vi "Window-Patches acq viewer (experimental).vi"() -> ()   [LabVIEW 2017]
uses:
  User Interface/Visualisation/Timelapse Viewer/Typedefs/Speed Viewer States enum.ctl
  User Interface/Visualisation/Timelapse Viewer/Typedefs/Time series viewer refs.ctl
  User Interface/Visualisation/Timelapse Viewer/Globals/gl_Time series viewer globals.vi
  User Interface/Visualisation/Timelapse Viewer/Typedefs/Select Play-Stop button to show.ctl
  <vilib>/Utility/miscctls.llb/LVPointTypeDef.ctl
  <vilib>/vision/Image Controls.llb/IMAQ Image.ctl
  User Interface/Visualisation/Timelapse Viewer/Cam video sync/Typedefs/Cam videos cluster.ctl
  User Interface/Visualisation/Functional Imaging Viewer/Typedefs/Get-Set-Clear Control.ctl
  <vilib>/Utility/error.llb/DialogType.ctl
  Typedefs/Save-Load enum.ctl
  User Interface/Visualisation/Timelapse Viewer/Typedefs/Custom slider-vertical.ctl
panel:
  in  "Speed chart history (sec)":i32=10
  out "Number of Frames":u32
  in  "Source number of frames":T1(ring)=enum."As many as the number of cycles"
  out "Cams":T3 {"Vid4 Rel time (ms)" format="%.0f ms"; "Vid3 Rel time (ms)" format="%.0f ms"; "Vid2 Rel time (ms)" format="%.0f ms"; "Vid1 Rel time (ms)" format="%.0f ms"}
  out "Original frame rate (fps)":dbl format="Original frame rate: %#.1f (fps)"
  out "Frame rate set (fps)":dbl format="Frame rate set: %#.1f (fps)"
  out "Actual frame rate (fps)":dbl format="Actual frame rate: %#.1f (fps)"
  out "AVI Mode ind":string="AVI mode:"
  out "Video length info":string="Duration: 00h 00m 00s, 0 frames"
  in  "Experiment path":path=path "C:/Users/Teo/Desktop/UCL Datasets/150501_13_00_36 SRINIVAS PATCHES"
  out "Export images":bool
  out "Export snippet":bool
  in  "Extraction Cursors":cluster{i32, i32}(slide)={1, 5594} scale=1.0..1950.0
  out "Export vid":bool
  out "Stop (ind)":bool
  in  "Intensity":T4={0.0, 4095.0} scale=0.0..4095.0
  out "Slider at frame #":i32 format="Slider at time-series frame: %.0f"
  in  "Scrollbar":i32(c297)
  in  "Back":bool
  in  "Play":bool
  in  "Stop":bool
  out "Actual number of speed points":i32 format="Actual of speed points: %.0f"
  out "Speed Data":string[][](array[string])
  out "Expected speed values":dbl format="Expected speed points: %#_g"
  in  "Colour":enum16{"Gray", "Red", "Green"}(ring)
  out "Image":T2(plugin-control)
  out "Speed Graph":dbl[](graph) caption="Speed Chart"
  # "This tool is under development.\nIt currently loads and displays cam videos and speed data acquired during functional acquisition experiments (POI/rectangles/volumes). It may be upgraded to visualise imaging data too."
  # "Timelapse Info"
  # "Date                         Time                  Time stamp           Speed (rpm)          Angle (deg)"
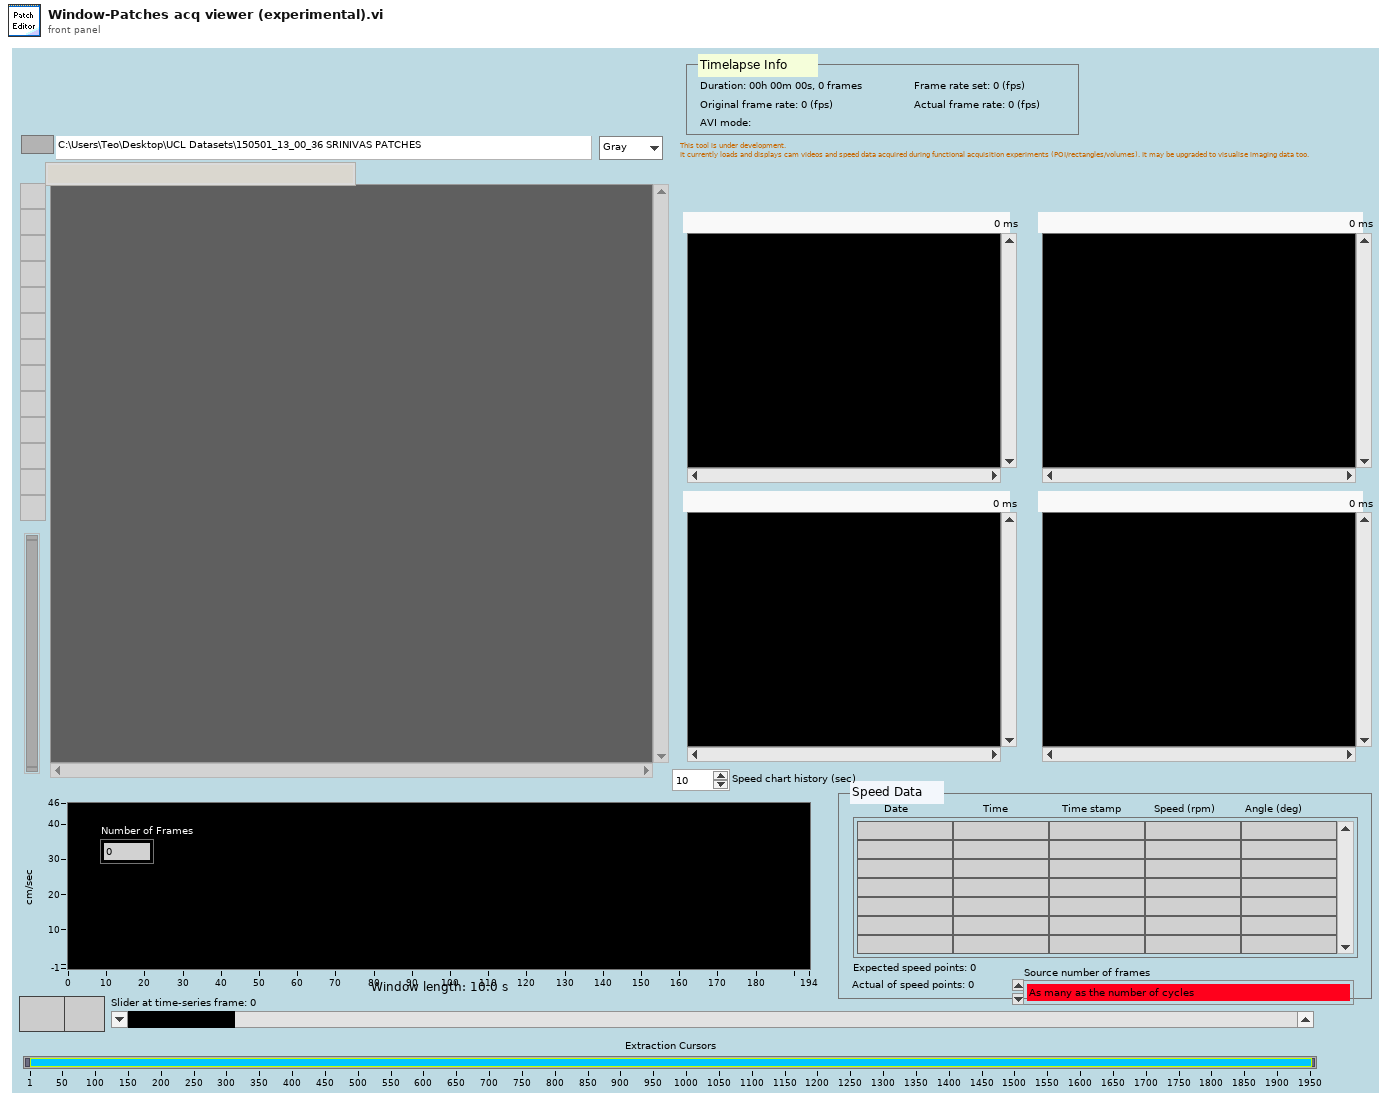
[diagram p1: front panel]
types:
  T1 = enum16{"As many as the frames in the video with the fewest frames", "As many as the number of cycles"}
  T2 = typedef "IMAQ Image.ctl" = refnum<image>
  T3 = cluster{"Vid 1":T2, "Vid 2":T2, "Vid 3":T2, "Vid 4":T2, "Vid1 Rel time (ms)":u32, "Vid2 Rel time (ms)":u32, "Vid3 Rel time (ms)":u32, "Vid4 Rel time (ms)":u32}
  T4 = typedef "Custom slider-vertical.ctl" = cluster{dbl, dbl}
  T5 = typedef "Time series viewer refs.ctl" = cluster{"This VI":refnum<vi>, "Image control":refnum<vi>, "AVI Mode ind":refnum<vi>, "Play":refnum<vi>, "Stop":refnum<vi>, "Back":refnum<vi>, "Scrollbar":refnum<vi>, "Video length info":refnum<vi>, "Expected speed values":refnum<vi>, "Intensity":refnum<vi>, "Path":refnum<vi>, "Selection sliders":refnum<vi>, "Speed Graph ref":refnum<vi>, "Frame rate set (fps)":refnum<vi>, "Channel to load":refnum<vi>, "Number of rows to generate":refnum<vi>, "Colour":refnum<vi>}
  T6 = typedef "Save-Load enum.ctl" = enum16{"Save to file", "Load from file", "Compare from file"}
  T7 = enum16{"None", "Release queue", "Obtain queue", "Enqueue", "Get status", "Set status"}
  T8 = typedef "LVPointTypeDef.ctl" = cluster{"Horizontal":i16, "Vertical":i16}
  T9 = typedef "Speed Viewer States enum.ctl" = enum16{"Idle", "Initialise", "Playback", "Scroll bar event", "Speed cursor event", "Back to start", "Exit"}
  T10 = typedef "Image Type" = u32
  T11 = typedef "IMAQ AVI2 Refnum.ctl" = refnum<k20>
  T12 = cluster{"# of frames to export":i32, "Initial frame's owning file":T11, "8-bit AVI file path":path, "Cursors location":cluster{"Number of first frame":i32, "Number of last frame":i32}}
  T13 = typedef "Get-Set-Clear Control.ctl" = enum16{"Get", "Set", "Clear"}
  T14 = typedef "Select Play-Stop button to show.ctl" = enum16{"Show Play button", "Show Stop button"}
  T15 = typedef "Cam videos cluster.ctl" = cluster{"Vid 1":T2, "Vid 2":T2, "Vid 3":T2, "Vid 4":T2, "Vid1 Rel time (ms)":u32, "Vid2 Rel time (ms)":u32, "Vid3 Rel time (ms)":u32, "Vid4 Rel time (ms)":u32}
  T16 = typedef "DialogType.ctl" = u16
  T17 = typedef "AVI modes refs cluster.ctl" = cluster{"AVI1 ref":T18, "AVI2 refs":T11[], "AVI # frames":u32[]}
  T18 = typedef "AviRefnum.ctl" = refnum<k1>
  T19 = typedef "AVI implementation enum.ctl" = enum16{"AVI1", "AVI2"}
  T20 = enum32{"Invalid", "Standard", "Closed", "Hidden", "Minimized", "Maximized"}
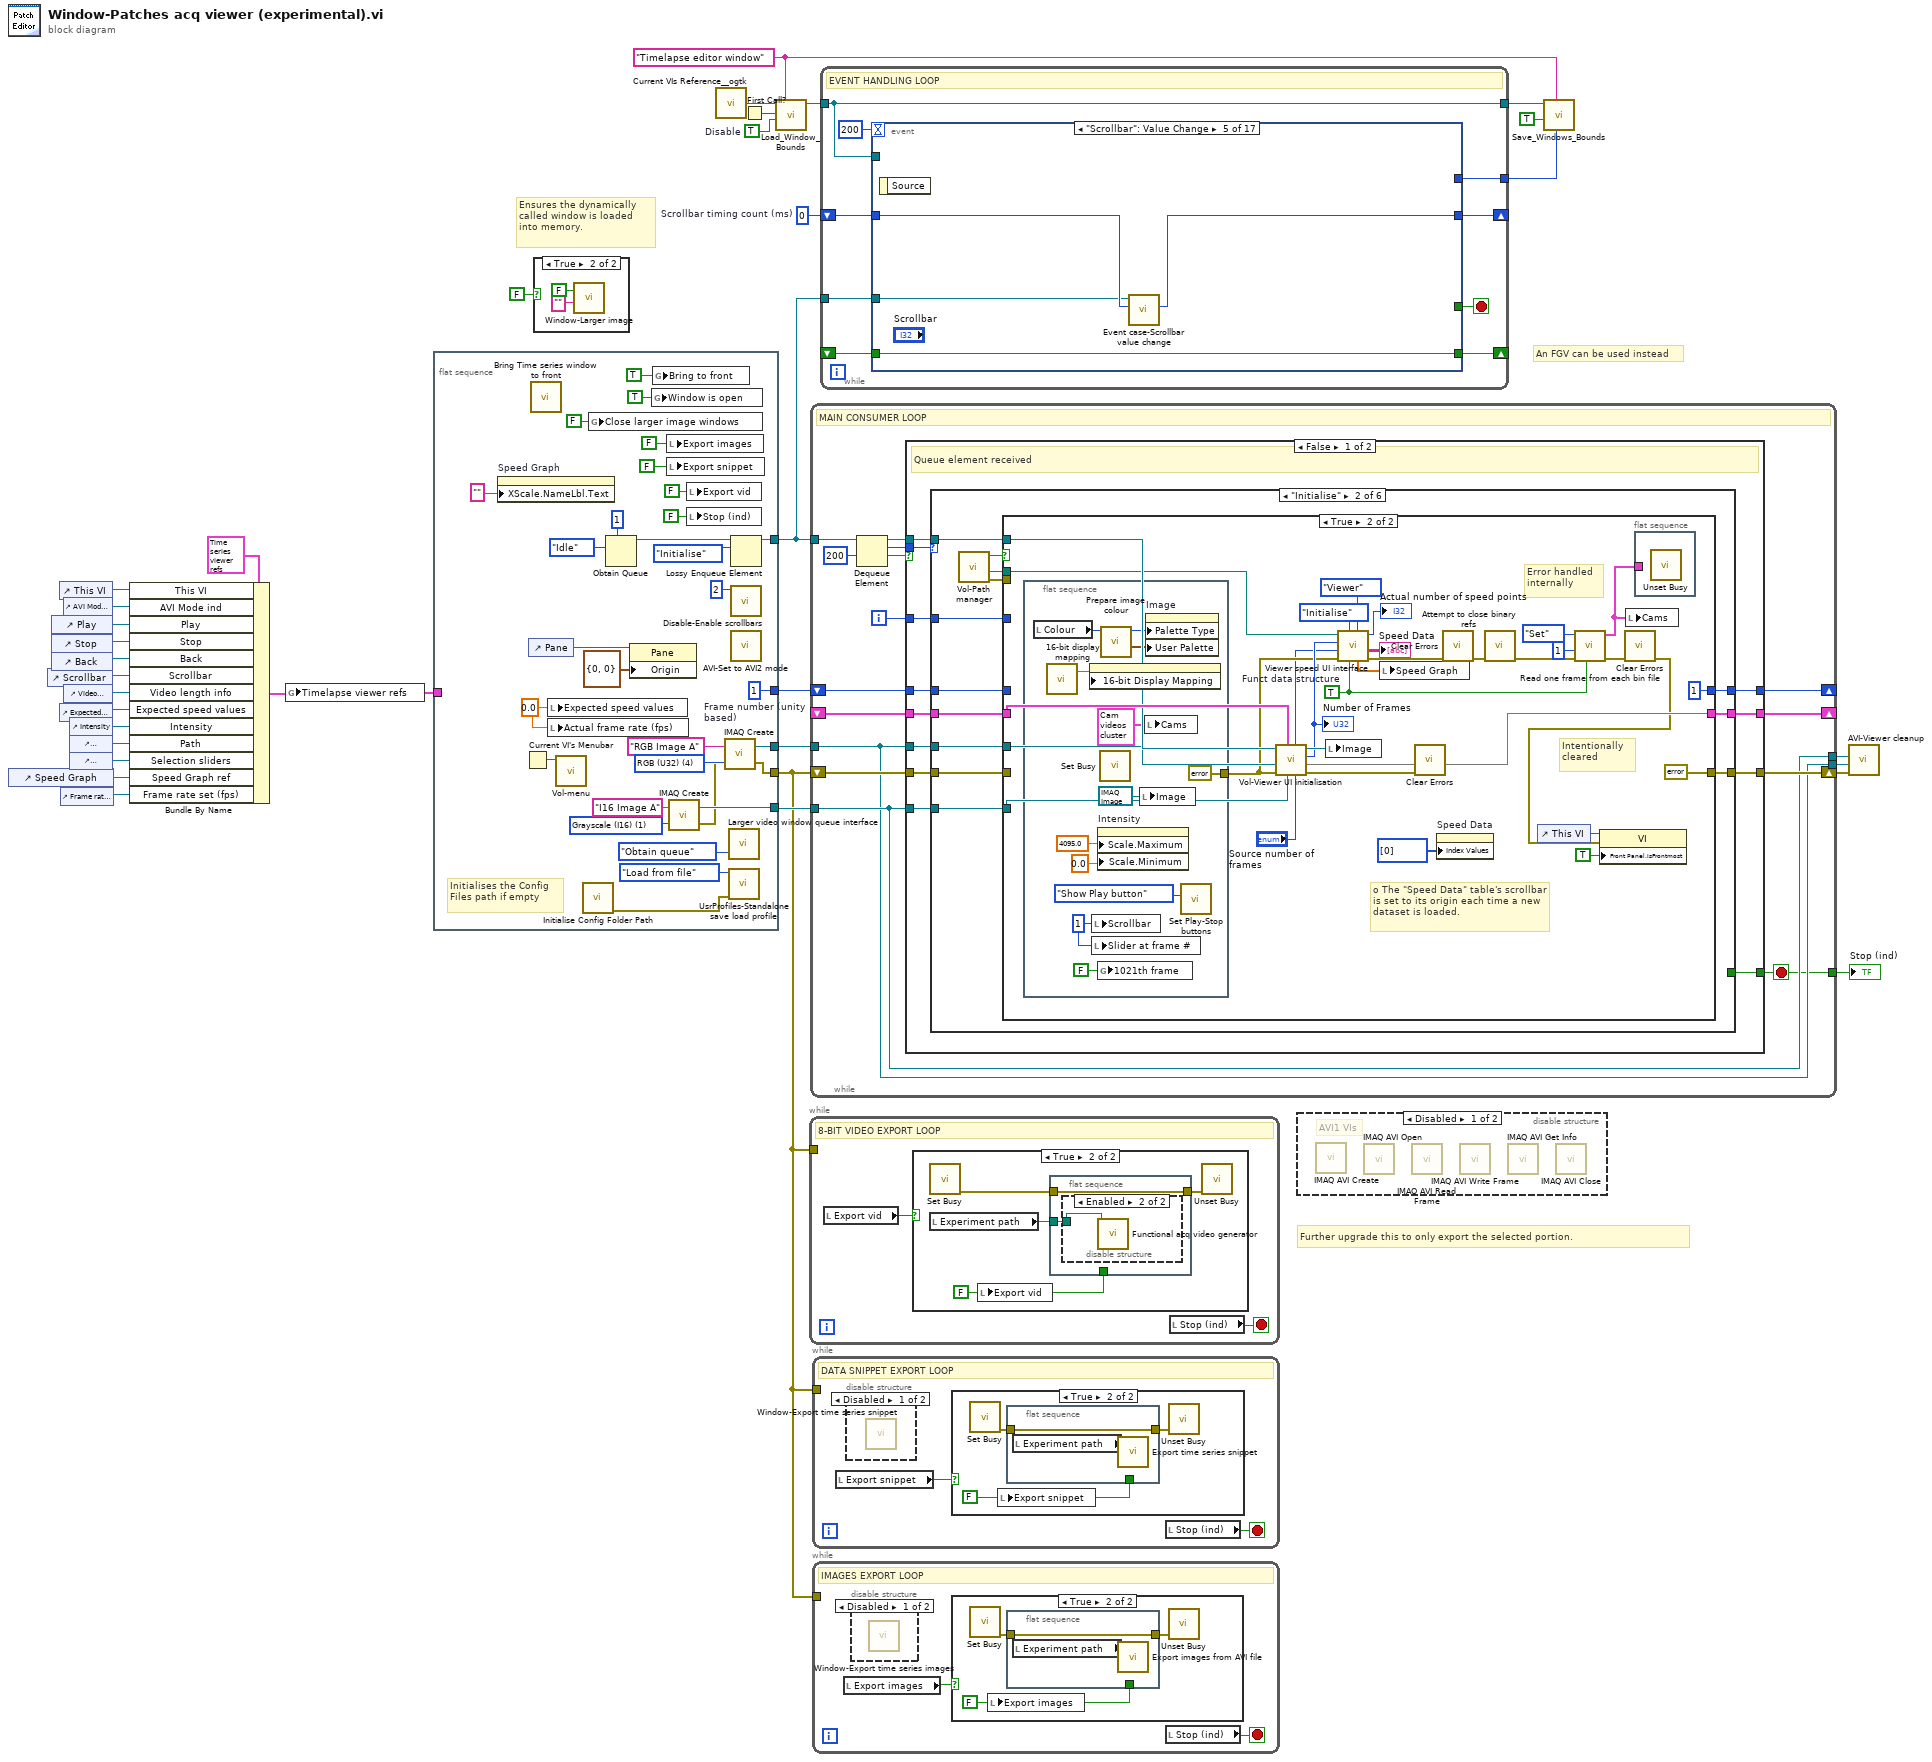
[diagram p0: block diagram]
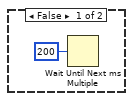
[diagram p4: hidden frame]
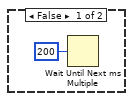
[diagram p6: hidden frame]
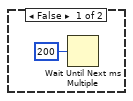
[diagram p8: hidden frame]
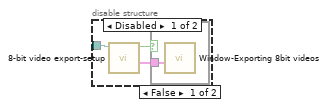
[diagram p9: hidden frame]
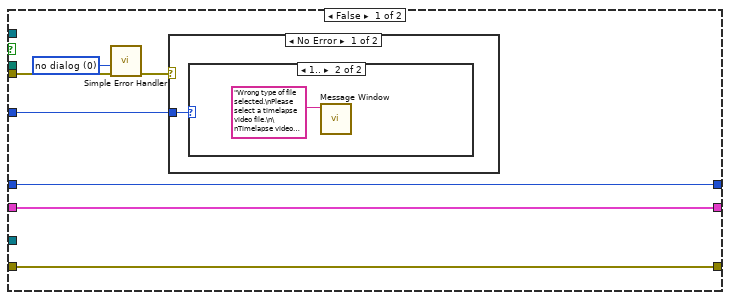
[diagram p12: hidden frame]
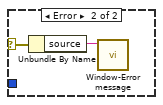
[diagram p14: hidden frame]
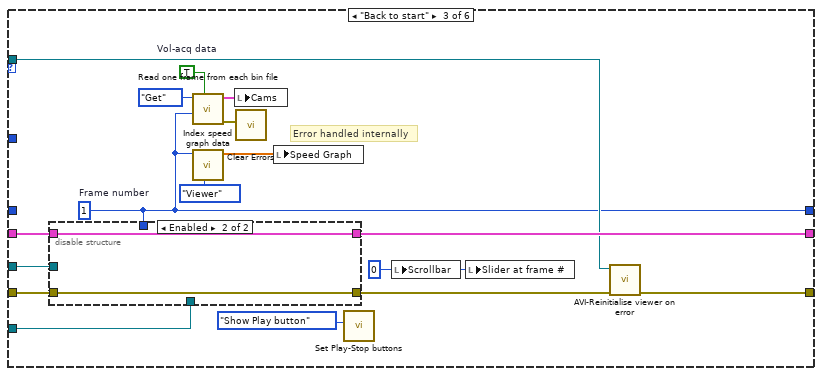
[diagram p15: hidden frame]
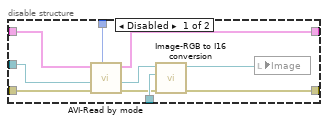
[diagram p16: hidden frame]
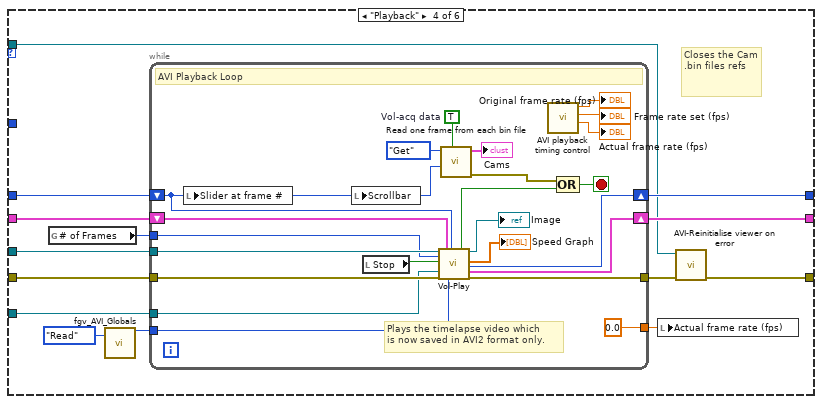
[diagram p17: hidden frame]
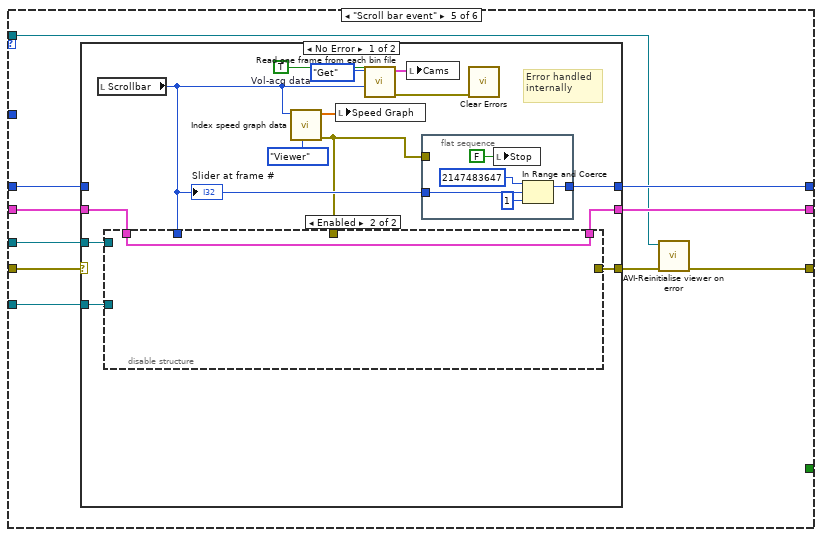
[diagram p18: hidden frame]
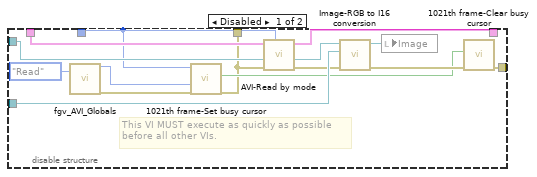
[diagram p19: hidden frame]
diagram:
  w10 = TRUE  # Disable
  w9 = "Timelapse editor window" ("Window Name (i.e. Key)")
  w2 = u32 0  # Scrollbar timing count (ms)
  # "Further upgrade this to only export the selected portion."
  # "Ensures the dynamically called window is loaded into memory."
  # "An FGV can be used instead"
  n1 = control-ref of="Speed Graph"() -> (w1:refnum<vi>)
  n2 = control-ref of="Scrollbar"() -> (w23:refnum<vi>)
  n3 = control-ref of="Play"() -> (w26:refnum<vi>)
  n4 = control-ref of="Stop"() -> (w25:refnum<vi>)
  n5 = control-ref of="Back"() -> (w24:refnum<vi>)
  n6 = control-ref of="This VI"() -> (w17:refnum<vi>)
  n7 = control-ref of="Expected speed values"() -> (w21:refnum<vi>)
  n8 = control-ref of="Frame rate set (fps)"() -> (w3:refnum<vi>)
  n9 = control-ref of="AVI Mode ind"() -> (w29:refnum<vi>)
  n10 = control-ref of="Video length info"() -> (w22:refnum<vi>)
  n11 = control-ref of="Intensity"() -> (w20:refnum<vi>)
  n12 = control-ref of="Experiment path"() -> (w19:refnum<vi>)
  n13 = control-ref of="Extraction Cursors"() -> (w14:refnum<vi>)
  n14 = Bundle By Name(cluster=T5 {"This VI"=refnum, "Image control"=refnum, "AVI Mode ind"=refnum, "Play"=refnum, "Stop"=refnum, "Back"=refnum, "Scrollbar"=refnum, "Video length info"=refnum, "Expected speed values"=refnum, "Intensity"=refnum, "Path"=refnum, "Selection sliders"=refnum, "Speed Graph ref"=refnum, "Frame rate set (fps)"=refnum, "Channel to load"=refnum, "Number of rows to generate"=refnum, "Colour"=refnum}, "This VI"=w17, "AVI Mode ind"=w29, "Play"=w26, "Stop"=w25, "Back"=w24, "Scrollbar"=w23, "Video length info"=w22, "Expected speed values"=w21, "Intensity"=w20, "Path"=w19, "Selection sliders"=w14, "Speed Graph ref"=w1, "Frame rate set (fps)"=w3) -> (w16:T5)
  n15 = global write "gl_Time series viewer globals.vi" "Timelapse viewer refs"(w16) -> ()
  n16 = flat-sequence {
    tunnel: [w62] -> w34
    tunnel: [w59] -> w33
    tunnel: [w51] -> w13
    tunnel: [w55] -> w31
    tunnel: [w53] -> w30
    tunnel: w16 -> [_]
    frame #0 {
      w48 = 0.0 ("Expected speed points")
      w53 = 1  # Frame number (unity based)
      w61 = T10 1 items=["Grayscale (U8)", "Grayscale (I16)", "Grayscale (SGL)", "Complex (CSG)", "RGB (U32)", "HSL (U32)", "RGB (U64)", "Grayscale (U16)"] ("Image Type")
      w63 = T10 4 items=["Grayscale (U8)", "Grayscale (I16)", "Grayscale (SGL)", "Complex (CSG)", "RGB (U32)", "HSL (U32)", "RGB (U64)", "Grayscale (U16)"] ("Image Type")
      # "Initialises the Config Files path if empty"
      n17 = property on="Speed Graph" class="WFGraph (strict)"("XScale.NameLbl.Text"="" ("X Scale.Name Label.Text")) -> ()  [unwired: 2 in, 2 out]
      n18 = Current VI's Menubar() -> (w47:refnum<k9>)
      n19 = control-ref of="Pane"() -> (w49:refnum<vi>)
      n20 = call "Bring Time series window to front.vi"() -> ()  [unwired: 12 in]
      n21 = local write "Expected speed values"(w48) -> ()
      n22 = local write "Actual frame rate (fps)"(w48) -> ()
      n23 = call "Vol-menu.vi"("menu"=w47) -> ()  [unwired: 9 in, 2 out]
      n24 = call "Initialise Config Folder Path.vi"() -> ("error out"=w36:errorcluster)  [unwired: 9 in, 2 out]
      n25 = global write "gl_Time series viewer globals.vi" "Close larger image windows"(FALSE ("Close larger image window")) -> ()
      n26 = Obtain Queue(max queue size (-1, unlimited)=1, element data type=Speed_Viewer_States_enum."Idle" ("States")) -> (queue out=w56:refnum<queue>)  [unwired: 3 in, 2 out]
      n27 = property class="Pane"(reference=w49, "Origin"=T8 {"Horizontal"=0, "Vertical"=0}) -> ()  [unwired: 1 in, 2 out]
      n28 = global write "gl_Time series viewer globals.vi" "Window is open"(TRUE ("Window is open")) -> ()
      n29 = global write "gl_Time series viewer globals.vi" "Bring to front"(TRUE ("Bring Timelapse Editor to front")) -> ()
      n30 = local write "Export images"(FALSE ("Export data subset")) -> ()
      n31 = local write "Export snippet"(FALSE ("Export data subset")) -> ()
      n32 = call "IMAQ Create"("Image Name"="I16 Image A", "Image Type"=w61) -> ("New Image"=w59:T2, "error out"=w52:errorcluster)  [unwired: 2 in, 1 out]
      n33 = local write "Export vid"(FALSE ("Export")) -> ()
      n34 = local write "Stop (ind)"(FALSE ("Boolean")) -> ()
      n35 = call "IMAQ Create"("Image Name"="RGB Image A", "Image Type"=w63, "error in (no error)"=w52) -> ("New Image"=w62:T2, "error out"=w51:errorcluster)  [unwired: 1 in, 1 out]
      n36 = call "Larger video window queue interface.vi"("Function"=T7."Obtain queue") -> ()  [unwired: 10 in, 1 out]
      n37 = call "UsrProfiles-Standalone save load profile.vi"("Error in"=w36, "Function"=Save-Load_enum."Load from file") -> ()  [unwired: 9 in, 1 out]
      n38 = Lossy Enqueue Element(queue=w56, element=Speed_Viewer_States_enum."Initialise" ("States")) -> (queue out=w55:refnum<queue>)  [unwired: 1 in, 3 out]
      n39 = call "Disable-Enable scrollbars.vi"("Disabled state"=2) -> ()  [unwired: 10 in, 1 out]
      n40 = call "AVI-Set to AVI2 mode.vi"() -> ()  [unwired: 11 in, 1 out]
    }
  }
  n41 = case shown="True" FALSE {
    frame False {
    }
    frame True {
      n42 = call "Window-Larger image.vi"("Image name"="", "Open maximised"=FALSE) -> ()  [unwired: 10 in]
    }
  }
  n43 = call <userlib>:"Current VIs Reference__ogtk.vi"() -> ("Current VI's reference"=w12:refnum<vi>)  [unwired: 5 in]
  n44 = First Call?() -> (First Call?: T/F=w11:bool)
  n45 = call "Load_Window_Bounds.vi"("Window Name (i.e. Key)"=w9, "Disable"=w10, "First Call"=w11, "Window VI's Ref"=w12) -> ("reference out"=w5:refnum<vi>)  [unwired: 4 in, 3 out]
  n46 = while {
    tunnel: w13 -> [_]
    stop <- w68 stop-if-true
    # "8-BIT VIDEO EXPORT LOOP"
    n47 = local read "Export vid"() -> (w67:bool)
    n48 = case shown="True" w67 {
      frame False {
        n49 = Wait Until Next ms Multiple(millisecond multiple=u32 200) -> ()  [unwired: 1 out]
      }
      frame True {
        w73 = FALSE ("Export")
        n50 = call <vilib>:"Set Busy.vi"() -> ("error out"=w72:errorcluster)  [unwired: 10 in, 1 out]
        n51 = local read "Experiment path"() -> (w70:path)
        n52 = local write "Export vid"(w73) -> ()
        n53 = flat-sequence {
          tunnel: w73 -> [_]
          tunnel: w72 -> [w75]
          tunnel: [w75] -> w71
          tunnel: w70 -> [w74]
          frame #0 {
            n54 = disable-structure shown="Enabled" {
              disable-tunnel: w74 -> [w76 w80]
              frame Disabled {
                n55 = call "8-bit video export-setup.vi"("Path"=w76) -> ("output cluster"=w78:T12, "cancelled"=w77:bool)  [unwired: 9 in]
                n56 = case shown="False" w77 {
                  tunnel: w78 -> [w79 _]
                  frame False {
                    n57 = call "Window-Exporting 8bit videos.vi"("Input cluster"=w79) -> ()  [unwired: 11 in]
                  }
                  frame True {
                  }
                }
              }
              frame Enabled {
                n58 = call "Functional acq video generator.vi"("ExperimentPath"=w80) -> ()  [unwired: 11 in]
              }
            }
          }
        }
        n59 = call <vilib>:"Unset Busy.vi"("error in (no error)"=w71) -> ()  [unwired: 10 in, 1 out]
      }
    }
    n60 = local read "Stop (ind)"() -> (w68:bool)
  }
  n61 = while {
    tunnel: w34 -> [w84]
    tunnel: w33 -> [w85]
    tunnel: [w85] -> w32
    shift-right: [w92] -> _
    shift-left: w30 -> [w91]
    tunnel: w31 -> [w90]
    shift-right: [w86] -> _
    shift-left: _ -> [w95]
    tunnel: [w84] -> w18
    shift-right: [w93] -> w27
    shift-left: w13 -> [w94]
    tunnel: [w82] -> w15
    i -> [w81]
    stop <- w82 stop-if-true
    # "MAIN CONSUMER LOOP"
    n62 = Dequeue Element(queue=w90, timeout in ms (-1)=200) -> (queue out=w83:refnum<queue>, element=w87:T9, timed out?=w88:bool)  [unwired: 1 in, 1 out]
    n63 = case shown="False" w88 {
      tunnel: w95 -> [w107 w305]
      tunnel: [w106 w305] -> w86
      tunnel: w84 -> [w105 _]
      tunnel: w85 -> [w104 _]
      tunnel: w94 -> [w103 w304]
      tunnel: [w102 w304] -> w93
      tunnel: [w101 w306] -> w92
      tunnel: w91 -> [w100 w306]
      tunnel: w87 -> [w99 _]
      tunnel: [w98 _] -> w82
      tunnel: w83 -> [w97 _]
      tunnel: w81 -> [w96 _]
      frame False {
        # "Queue element received"
        n64 = case shown="\"Initialise\"" w99 {
          tunnel: w107 -> [w109 w123 w193 w220 w249 w294]
          tunnel: [w109 w119 w192 w214 w251 w294] -> w106
          tunnel: w105 -> [_ w118 w190 w219 w250 _]
          tunnel: w104 -> [_ w117 w191 w218 w253 _]
          tunnel: w103 -> [w108 w121 w189 w217 w248 w293]
          tunnel: [w108 w120 w186 w213 w246 w292] -> w102
          tunnel: [w110 w122 w183 w216 w252 1 ("Slide")] -> w101
          tunnel: w100 -> [w110 w116 _ w215 w247 _]
          tunnel: [_ _ _ _ _ TRUE] -> w98
          tunnel: w97 -> [_ w112 w185 w211 w244 _]
          tunnel: w96 -> [_ w111 _ _ _ _]
          frame Default {
          }
          frame "Initialise" {
            n65 = call "Vol-Path manager.vi"() -> ("error"=w113:errorcluster, "Speed Data folder path+dummy filename"=w114:path, "File path OK"=w115:bool)  [unwired: 9 in]
            n66 = case shown="True" w115 {
              tunnel: w123 -> [w129 w165]
              tunnel: [w130 1] -> w122
              tunnel: w114 -> [_ w148]
              tunnel: w121 -> [w128 _]
              tunnel: [w128 errorcluster {"status"=FALSE, "code"=0, "source"=""} ("error out")] -> w120
              tunnel: [w129 w157] -> w119
              tunnel: w118 -> [_ w156]
              tunnel: w117 -> [_ w163]
              tunnel: w116 -> [w130 _]
              tunnel: w113 -> [w127 _]
              tunnel: w112 -> [_ w160]
              tunnel: w111 -> [w124 _]
              frame False {
                w126 = T16 0 items=["no dialog", "OK message", "continue or stop message", "OK message + warnings", "continue/stop + warnings"] ("type of dialog (OK msg:1)")
                n67 = call <vilib>:"Simple Error Handler.vi"("type of dialog (OK msg:1)"=w126, "error in (no error)"=w127) -> ("error out"=w125:errorcluster)  [unwired: 3 in, 4 out]
                n68 = case shown="No Error" w125 {
                  selector: w125 -> [_ w134]
                  tunnel: w124 -> [w131 _]
                  frame No Error {
                    n69 = case shown="1.." w131 {
                      frame 0, Default {
                      }
                      frame 1.. {
                        n70 = call "Message Window.vi"("Message string"="Wrong type of file selected.\nPlease select a timelapse video file.\n\nTimelapse video files are located  in timelapse folders \ne.g. \"TimeLapse 02_10_2014 20-22-02\"\nand their file names are similar to this: \"Green Channel 1\"\n\nNote: For timelapse video files which are part of a split-files sequence e.g. Green Channel 1, Green Channel 2, Green Channel 3... \ndouble click on any one file. The full sequence will open in the viewer regardless of which file you select.") -> ()  [unwired: 10 in, 1 out]
                      }
                    }
                  }
                  frame Error {
                    n71 = Unbundle By Name(w134) -> ("source"=w133:string)
                    n72 = call "Window-Error message.vi"("Message"=w133) -> ()  [unwired: 10 in, 1 out]
                  }
                }
              }
              frame True {
                w138 = TRUE  # Funct data structure
                # "o\tThe \"Speed Data\" table's scrollbar is set to its origin each time a new dataset is loaded."
                # "Error handled internally"
                # "Intentionally cleared"
                n73 = flat-sequence {
                  tunnel: [errorcluster {"status"=FALSE, "code"=0, "source"=""} ("error out")] -> w149
                  frame #0 {
                    w166 = 1 ("Scrollbar")
                    n74 = local read "Colour"() -> (w174:enum16{"Gray", "Red", "Green"})
                    n75 = call "16-bit display mapping.vi"() -> (2:w171)  [unwired: 10 in, 1 out]
                    n76 = property on="Image" class="ImageControl"("16-bit Display Mapping"=w171) -> ()  [unwired: 2 in, 2 out]
                    n77 = local write "Scrollbar"(w166) -> ()
                    n78 = local write "Slider at frame #"(w166) -> ()
                    n79 = property on="Intensity" class="Slide (strict)"("Scale.Maximum"=4095.0 ("Scale.Range:Maximum"), "Scale.Minimum"=0.0 ("Scale.Range:Minimum")) -> ()  [unwired: 2 in, 2 out]
                    n80 = global write "gl_Time series viewer globals.vi" "1021th frame"(FALSE ("1021th frame")) -> ()
                    n81 = call <vilib>:"Set Busy.vi"() -> ()  [unwired: 10 in, 2 out]
                    n82 = call "Prepare image colour.vi"("Left Image Palette"=w174) -> ("Color Palette"=w172:cluster{"Red":u8, "Green":u8, "Blue":u8}[], "Palette Type"=w173:u32)  [unwired: 8 in, 1 out]
                    n83 = local write "Image"(T2 refnum ("New Image")) -> ()
                    n84 = local write "Cams"(T15 {"Vid 1"=refnum, "Vid 2"=refnum, "Vid 3"=refnum, "Vid 4"=refnum, "Vid1 Rel time (ms)"=0, "Vid2 Rel time (ms)"=0, "Vid3 Rel time (ms)"=0, "Vid4 Rel time (ms)"=0} ("Cam videos cluster")) -> ()
                    n85 = property on="Image" class="ImageControl"("Palette Type"=w173, "User Palette"=w172) -> ()  [unwired: 2 in, 2 out]
                    n86 = call "Set Play-Stop buttons.vi"("Function"=Select_Play-Stop_button_to_show."Show Play button") -> ()  [unwired: 10 in, 1 out]
                  }
                }
                n87 = call "Vol-Viewer UI initialisation.vi"("Source number of frames"="Source number of frames", 6:w163, 7:w165, "error in (no error)"=w149, 9:w156, 11:w160) -> ("error out"=w161:errorcluster, 1:w157, "Number of Frames"=w158:u32, "Image ref"=w159:T2, "Scrollbar position"=w137:i32)  [unwired: 1 in]
                "Number of Frames" <- w158
                n88 = local write "Image"(w159) -> ()
                n89 = call "Viewer speed UI interface.vi"("Caller"=enum16{"Viewer", "Exporter"}."Viewer", "Funct data structure"=w138, "Function"=enum16{"Initialise", "Update"}."Initialise", "error in (no error)"=w149, "Gobal frame number in Timelapse data/master video (1 based)"=w137, "Number of Frames"=w158, "Speed Data folder path+dummy filename"=w148) -> ("error out"=w154:errorcluster, "Speed Data"=→"Speed Data":string[][], "Actual number of speed values"=→"Actual number of speed points":i32, "Speed waveform graph data"=w136:dbl[])  [unwired: 1 in]
                n90 = local write "Speed Graph"(w136) -> ()
                n91 = call <vilib>:"Clear Errors.vi"("error in (no error)"=w161) -> ()  [unwired: 5 in, 2 out]
                n92 = property on="Speed Data" class="Arr (strict)"("Index Values"=u32[] [0]) -> ()  [unwired: 2 in, 2 out]
                n93 = call <vilib>:"Clear Errors.vi"("error in (no error)"=w154) -> ("error out"=w150:errorcluster)  [unwired: 5 in, 1 out]
                n94 = call "Attempt to close binary refs.vi"("error in (no error)"=w150) -> ("error out"=w151:errorcluster)  [unwired: 10 in]
                n95 = control-ref of="This VI"() -> (w142:refnum<vi>)
                n96 = call "Read one frame from each bin file.vi"("Funct data structure"=w138, "error in (no error)"=w151, "Master video's frame number (unity-based)"=1 ("Frame number"), "Get/set"=Get-Set-Clear_Control."Set" ("GEt set .bin refs")) -> ("Error out"=w146:errorcluster, "Cam videos cluster"=w147:T15)  [unwired: 6 in]
                n97 = call <vilib>:"Clear Errors.vi"("error in (no error)"=w146) -> ("error out"=w140:errorcluster)  [unwired: 5 in, 1 out]
                n98 = property on="Property Node" class="VI"(reference=w142, error in=w140, "Front Panel.IsFrontmost"=TRUE ("Front Panel Window:Is Frontmost")) -> ()  [unwired: 2 out]
                n99 = local write "Cams"(w147) -> ()
                n100 = flat-sequence {
                  tunnel: w147 -> [_]
                  frame #0 {
                    n101 = call <vilib>:"Unset Busy.vi"() -> ()  [unwired: 11 in, 1 out]
                  }
                }
              }
            }
          }
          frame "Back to start" {
            w180 = TRUE  # Vol-acq data
            w194 = 0 ("Scrollbar")
            w183 = 1  # Frame number
            # "Error handled internally"
            n102 = disable-structure shown="Enabled" {
              disable-tunnel: w193 -> [w203 w206]
              disable-tunnel: [w202 w206] -> w192
              disable-tunnel: w191 -> [w201 _]
              disable-tunnel: w190 -> [w200 _]
              disable-tunnel: w189 -> [w198 w205]
              disable-tunnel: [w196 w205] -> w187
              disable-tunnel: w183 -> [w195 _]
              frame Disabled {
                n103 = call "AVI-Read by mode.vi"("Frame number (unity-based)"=w195, "error in (no error)"=w198, "RGB image ref in"=w200, "AVI modes refs"=w203) -> ("error out"=w197:errorcluster, "RGB image ref out"=w204:T2, "AVI modes refs"=w202:T17)  [unwired: 5 in]
                n104 = call "Image-RGB to I16 conversion.vi"("error in (no error)"=w197, "I16 image ref in"=w201, "RGB image ref in"=w204) -> ("error out"=w196:errorcluster, "I16 image ref out"=w199:T2)  [unwired: 7 in]
                n105 = local write "Image"(w199) -> ()
              }
              frame Enabled {
              }
            }
            n106 = call "Read one frame from each bin file.vi"("Funct data structure"=w180, "Master video's frame number (unity-based)"=w183, "Get/set"=Get-Set-Clear_Control."Get" ("GEt set .bin refs")) -> ("Error out"=w181:errorcluster, "Cam videos cluster"=w184:T15)  [unwired: 7 in]
            n107 = call "Index speed graph data.vi"("Caller"=enum16{"Viewer", "Exporter"}."Viewer", "Gobal frame number in Timelapse data/master video (1 based)"=w183) -> ("Speed data waveform graph"=w179:dbl[])  [unwired: 7 in, 2 out]
            n108 = local write "Cams"(w184) -> ()
            n109 = call <vilib>:"Clear Errors.vi"("error in (no error)"=w181) -> ()  [unwired: 5 in, 2 out]
            n110 = local write "Speed Graph"(w179) -> ()
            n111 = call "Set Play-Stop buttons.vi"("Function"=Select_Play-Stop_button_to_show."Show Play button") -> ()  [unwired: 10 in, 1 out]
            n112 = local write "Scrollbar"(w194) -> ()
            n113 = local write "Slider at frame #"(w194) -> ()
            n114 = call "AVI-Reinitialise viewer on error.vi"("error in (no error)"=w187, "Queue in"=w185) -> ("error out"=w186:errorcluster)  [unwired: 9 in]
          }
          frame "Playback" {
            # "Closes the Cam .bin files refs"
            n115 = global read "gl_Time series viewer globals.vi" "# of Frames"() -> (w208:u32)
            n116 = call "fgv_AVI_Globals.vi"("Function"=enum16{"Intialize", "Write", "Read", "Clear"}."Read") -> ("AVI mode"=w209:T19)  [unwired: 11 in, 3 out]
            n117 = while {
              tunnel: w219 -> [w241]
              tunnel: w218 -> [w232]
              tunnel: w217 -> [w239]
              tunnel: [w240] -> w212
              shift-right: [w238] -> w216
              shift-left: w215 -> [w227]
              shift-right: [w242] -> w214
              shift-left: w220 -> [w243]
              tunnel: w209 -> [w234]
              tunnel: w208 -> [w231]
              tunnel: [0.0 ("Expected speed points")] -> w207
              stop <- w224 stop-if-true
              w222 = TRUE  # Vol-acq data
              # "Plays the timelapse video which \nis now saved in AVI2 format only."
              # "AVI Playback Loop"
              n118 = local write "Slider at frame #"(w227) -> ()
              n119 = local write "Scrollbar"(w227) -> ()
              n120 = local read "Stop"() -> (w233:bool)
              n121 = call "Vol-Play.vi"("RGB Image ref"=w241, "Number of Frames"=w231, "Stop button pressed"=w233, "I16 Image ref"=w232, "error in (no error)"=w239, "AVI modes refs in"=w243, "AVI mode"=w234, "Frame number (in)"=w227) -> ("Playback stopped"=w225:bool, "I16 image ref out"=→"Image":T2, "Speed data waveform graph"=→"Speed Graph":dbl[], "Frame number (out)"=w238:i32, "AVI modes refs out"=w242:T17, "error out"=w240:errorcluster)  [unwired: 6 in]
              n122 = call "Read one frame from each bin file.vi"("Funct data structure"=w222, "Master video's frame number (unity-based)"=w227, "Get/set"=Get-Set-Clear_Control."Get" ("GEt set .bin refs")) -> ("Error out"=w223:errorcluster, "Cam videos cluster"=→"Cams":T15)  [unwired: 7 in]
              n123 = call "AVI playback timing control.vi"() -> ("Actual frame rate (fps)"=→"Actual frame rate (fps)":dbl, "Frame rate set OR original (fps)"=→"Frame rate set (fps)":dbl, "Original frame rate (fps)"=→"Original frame rate (fps)":dbl)  [unwired: 8 in, 1 out]
              n124 = Compound Arithmetic op=OR(w223, w225) -> (w224:bool)
            }
            n125 = local write "Actual frame rate (fps)"(w207) -> ()
            n126 = call "AVI-Reinitialise viewer on error.vi"("error in (no error)"=w212, "Queue in"=w211) -> ("error out"=w213:errorcluster)  [unwired: 9 in]
          }
          frame "Scroll bar event" {
            n127 = case shown="No Error" w248 {
              selector: w248 -> [_ w291]
              tunnel: w253 -> [w267 _]
              tunnel: [w266 w290] -> w252
              tunnel: [w262 w289] -> w251
              tunnel: w250 -> [w265 _]
              tunnel: w249 -> [w264 w289]
              tunnel: [w263 w291] -> w245
              tunnel: w247 -> [_ w290]
              frame No Error {
                w256 = TRUE  # Vol-acq data
                # "Error handled internally"
                n128 = local read "Scrollbar"() -> (w258:i32)
                "Slider at frame #" <- w258
                n129 = disable-structure shown="Enabled" {
                  disable-tunnel: w267 -> [w282 _]
                  disable-tunnel: w265 -> [w279 _]
                  disable-tunnel: w264 -> [w277 w283]
                  disable-tunnel: [w272 _] -> w263
                  disable-tunnel: [w270 w283] -> w262
                  disable-tunnel: w258 -> [w269 _]
                  disable-tunnel: [w268 _] -> w257
                  frame Disabled {
                    # "This VI MUST execute as quickly as possible\nbefore all other VIs."
                    n130 = call "fgv_AVI_Globals.vi"("Function"=enum16{"Intialize", "Write", "Read", "Clear"}."Read") -> ("AVI mode"=w275:T19, "error out"=w274:errorcluster)  [unwired: 11 in, 2 out]
                    n131 = call "1021th frame-Set busy cursor.vi"("error in (no error)"=w274, "AVI mode"=w275, "Frame number"=w269) -> ("error out"=w268:errorcluster, "Busy cursor was set"=w271:bool)  [unwired: 7 in]
                    n132 = call "AVI-Read by mode.vi"("Frame number (unity-based)"=w269, "error in (no error)"=w268, "RGB image ref in"=w279, "AVI modes refs"=w277) -> ("error out"=w280:errorcluster, "RGB image ref out"=w278:T2, "AVI modes refs"=w270:T17)  [unwired: 5 in]
                    n133 = call "Image-RGB to I16 conversion.vi"("error in (no error)"=w280, "I16 image ref in"=w282, "RGB image ref in"=w278) -> ("error out"=w273:errorcluster, "I16 image ref out"=w281:T2)  [unwired: 7 in]
                    n134 = local write "Image"(w281) -> ()
                    n135 = call "1021th frame-Clear busy cursor.vi"("error in (no error)"=w273, "Busy cursor was set"=w271) -> ("error out"=w272:errorcluster)  [unwired: 9 in]
                  }
                  frame Enabled {
                  }
                }
                n136 = call "Index speed graph data.vi"("Caller"=enum16{"Viewer", "Exporter"}."Viewer", "error in (no error)"=w257, "Gobal frame number in Timelapse data/master video (1 based)"=w258) -> ("Speed data waveform graph"=w255:dbl[])  [unwired: 6 in, 2 out]
                n137 = local write "Speed Graph"(w255) -> ()
                n138 = call "Read one frame from each bin file.vi"("Funct data structure"=w256, "Master video's frame number (unity-based)"=w258, "Get/set"=Get-Set-Clear_Control."Get" ("GEt set .bin refs")) -> ("Error out"=w259:errorcluster, "Cam videos cluster"=w261:T15)  [unwired: 7 in]
                n139 = local write "Cams"(w261) -> ()
                n140 = flat-sequence {
                  tunnel: [w286] -> w266
                  tunnel: w258 -> [w284]
                  tunnel: w257 -> [_]
                  frame #0 {
                    n141 = local write "Stop"(FALSE ("Stop")) -> ()
                    n142 = In Range and Coerce(upper limit=2147483647, x=w284, lower limit=1) -> (coerced(x)=w286:i32)  [unwired: 1 out]
                  }
                }
                n143 = call <vilib>:"Clear Errors.vi"("error in (no error)"=w259) -> ()  [unwired: 5 in, 2 out]
              }
              frame Error {
              }
            }
            n144 = call "AVI-Reinitialise viewer on error.vi"("error in (no error)"=w245, "Queue in"=w244) -> ("error out"=w246:errorcluster)  [unwired: 9 in]
          }
          frame "Exit" {
            n145 = disable-structure shown="Enabled" {
              disable-tunnel: w294 -> [w300 _]
              disable-tunnel: w293 -> [w299 w302]
              disable-tunnel: [w298 w302] -> w292
              frame Disabled {
                n146 = Unbundle By Name(w300) -> ("AVI2 refs"=w301:T11[])
                n147 = call "AVI-AVI2 Close all.vi"("error in (no error)"=w299, "AVI2 ref"=w301) -> ("error out"=w298:errorcluster)  [unwired: 9 in]
              }
              frame Enabled {
              }
            }
            n148 = local read "Stop"() -> (w297:bool)
            n149 = case shown="True" w297 {
              frame False {
              }
              frame True {
                n150 = local write "Stop"(FALSE ("Stop")) -> ()
              }
            }
          }
        }
      }
      frame True {
        # "Timeout"
      }
    }
  }
  "Stop (ind)" <- w15
  n151 = while {
    tunnel: w13 -> [_]
    stop <- w308 stop-if-true
    # "DATA SNIPPET EXPORT LOOP"
    n152 = local read "Export snippet"() -> (w307:bool)
    n153 = disable-structure shown="Disabled" {
      frame Disabled {
        n154 = call "Window-Export time series snippet.vi"() -> ()  [unwired: 12 in]
      }
      frame Enabled {
      }
    }
    n155 = case shown="True" w307 {
      frame False {
        n156 = Wait Until Next ms Multiple(millisecond multiple=u32 200) -> ()  [unwired: 1 out]
      }
      frame True {
        w312 = FALSE ("Export data subset")
        n157 = call <vilib>:"Set Busy.vi"() -> ("error out"=w311:errorcluster)  [unwired: 10 in, 1 out]
        n158 = local write "Export snippet"(w312) -> ()
        n159 = flat-sequence {
          tunnel: w312 -> [_]
          tunnel: w311 -> [w314]
          tunnel: [w314] -> w310
          frame #0 {
            n160 = local read "Experiment path"() -> (w313:path)
            n161 = call "Export time series snippet.vi"("AVI File Path"=w313) -> ()  [unwired: 11 in]
          }
        }
        n162 = call <vilib>:"Unset Busy.vi"("error in (no error)"=w310) -> ()  [unwired: 10 in, 1 out]
      }
    }
    n163 = local read "Stop (ind)"() -> (w308:bool)
  }
  n164 = while {
    tunnel: w13 -> [_]
    stop <- w316 stop-if-true
    # "IMAGES EXPORT LOOP"
    n165 = local read "Export images"() -> (w315:bool)
    n166 = disable-structure shown="Disabled" {
      frame Disabled {
        n167 = call "Window-Export time series images.vi"() -> ()  [unwired: 12 in]
      }
      frame Enabled {
      }
    }
    n168 = case shown="True" w315 {
      frame False {
        n169 = Wait Until Next ms Multiple(millisecond multiple=u32 200) -> ()  [unwired: 1 out]
      }
      frame True {
        w318 = FALSE ("Export data subset")
        n170 = call <vilib>:"Set Busy.vi"() -> ("error out"=w320:errorcluster)  [unwired: 10 in, 1 out]
        n171 = local write "Export images"(w318) -> ()
        n172 = flat-sequence {
          tunnel: w318 -> [_]
          tunnel: w320 -> [w322]
          tunnel: [w322] -> w319
          frame #0 {
            n173 = local read "Experiment path"() -> (w321:path)
            n174 = call "Export images from AVI file.vi"("AVI File Path"=w321) -> ()  [unwired: 11 in]
          }
        }
        n175 = call <vilib>:"Unset Busy.vi"("error in (no error)"=w319) -> ()  [unwired: 10 in, 1 out]
      }
    }
    n176 = local read "Stop (ind)"() -> (w316:bool)
  }
  n177 = while {
    shift-right: [w329] -> _
    shift-left: w2 -> [w328]
    tunnel: w31 -> [w327]
    shift-right: [w326] -> _
    shift-left: _ -> [w325]
    tunnel: [w324] -> w4
    tunnel: w5 -> [w323]
    tunnel: [w323] -> w6
    stop <- w330 stop-if-true
    # "EVENT HANDLING LOOP"
    n178 = event shown="[4] \"Scrollbar\": Value Change" {
      selector: _ -> [_ _ _ _ _ _ _ _ _ _ _ _ _ _ _ _ _]
      dyn-events: _ -> [_ _ _ _ _ _ _ _ _ _ _ _ _ _ _ _ _]
      timeout: 200 -> [_ _ _ _ _ _ _ _ _ _ _ _ _ _ _ _ _]
      tunnel: [_ w337 _ _ _ _ _ _ _ _ _ _ _ _ _ _ w436] -> w330
      tunnel: [w335 w340 w353 w356 w358 w371 w385 w390 w392 w397 w405 w410 w415 w418 w423 w431 w438] -> w329
      tunnel: w328 -> [w335 w340 w353 w356 w360 w373 w385 w390 w392 w397 w405 w410 w415 w418 w423 w431 w438]
      tunnel: w327 -> [_ w338 _ _ w359 w372 _ w389 _ _ _ _ w412 _ w422 _ w437]
      tunnel: [w334 w336 w352 w355 w357 w362 w381 w387 w391 w393 FALSE FALSE w411 w416 w419 w430 w435] -> w326
      tunnel: w325 -> [w334 w336 w352 w355 w357 w362 w381 w387 w391 _ w404 _ w411 w416 w419 w430 w435]
      tunnel: [w332 _ _ _ _ _ _ _ _ _ _ _ _ _ _ _ w434] -> w324
      tunnel: w323 -> [w333 _ _ _ _ _ _ _ _ _ _ _ _ _ _ _ w433]
      event Timeout {
        n179 = event-data() -> ()  [unwired: 1 in, 1 out]
        n180 = call "Bring Time series window to front.vi"() -> ()  [unwired: 12 in]
        n181 = property class="VI"(reference=w333) -> ("FP.State"=w332:T20)  [unwired: 1 in, 2 out]
      }
      event Menu Selection (User) {
        n182 = event-data() -> ("ItemTag"=w339:string)  [unwired: 1 in]
        n183 = case shown="\"Export 8-bit video\"" w339 {
          tunnel: w338 -> [_ w341 _ _ w346 _ _ _]
          tunnel: [_ _ _ _ w345 _ _ _] -> w337
          frame Default {
          }
          frame "Load dataset" {
            n184 = call "Vol-Event handler-Load dataset.vi"("queue"=w341) -> ()  [unwired: 11 in]
          }
          frame "Playback speed..." {
            n185 = call "Window-Playback speed entry.vi"() -> ("Frame rate set (fps)"=w342:dbl)  [unwired: 10 in, 1 out]
            n186 = local write "Frame rate set (fps)"(w342) -> ()
          }
          frame "Original speed (x1)" {
            n187 = flat-sequence {
              frame #0 {
                n188 = global write "gl_Time series viewer globals.vi" "Use manual FPS?"(FALSE ("Use manual FPS?")) -> ()
              }
              frame #1 {
                n189 = call "AVI playback timing control.vi"() -> ("Frame rate set OR original (fps)"=w344:dbl)  [unwired: 8 in, 3 out]
                n190 = local write "Frame rate set (fps)"(w344) -> ()
              }
            }
          }
          frame "Close" {
            n191 = call "Time series viewer-Event handler-Exit.vi"("Queue in"=w346) -> ("Exit"=w345:bool)  [unwired: 10 in]
            n192 = case shown="True" w345 {
              frame False {
              }
              frame True {
                n193 = local write "Stop"(TRUE ("Stop")) -> ()
              }
            }
          }
          frame "Export snippet" {
            "Export snippet" <- TRUE
          }
          frame "Export 8-bit video" {
            "Export vid" <- TRUE
          }
          frame "Export TIFF series" {
            "Export images" <- TRUE
          }
        }
      }
      event "Scrollbar", "Speed Graph": Shortcut Menu Selection (User) {
        n194 = event-data() -> ("ItemTag"=w351:string)  [unwired: 1 in, 1 out]
        n195 = call "Time series viewer-Shortcut menu handler.vi"("ItemTag"=w351) -> ()  [unwired: 11 in]
      }
      event "Speed Graph": event type 3.0.x80000027 {
        n196 = event-data() -> ()  [unwired: 1 in, 1 out]
        n197 = event-data("Discard?"=TRUE) -> ()  [unwired: 1 in, 1 out]
      }
      event "Scrollbar": Value Change {
        n198 = event-data() -> ()  [unwired: 1 in, 1 out]
        n199 = call "Event case-Scrollbar value change.vi"("Tick count in"=w360, "Queue in"=w359) -> ("Tick count"=w358:u32)  [unwired: 8 in, 1 out]
      }
      event "Extraction Cursors": Value Change {
        # "Sets the main slider to the value of the extraction cursor that was moved."
        n200 = event-data() -> ("OldVal"=w370:cluster{i32, i32}, "NewVal"=w363:cluster{i32, i32})  [unwired: 1 in]
        n201 = Not Equal?(x=w370, y=w363) -> (x != y?=w364:cluster{bool, bool})
        n202 = Unbundle(w364) -> (w361:bool)  [unwired: 1 out]
        n203 = Unbundle(w363) -> (w369:i32, w368:i32)
        n204 = Select(t=w368, s=w361, f=w369) -> (s? t:f=w365:i32)
        n205 = flat-sequence {
          tunnel: w372 -> [w376]
          tunnel: w373 -> [w377]
          tunnel: [w377] -> w367
          tunnel: [w376] -> w366
          tunnel: w365 -> [w375]
          tunnel: w361 -> [w374]
          tunnel: [w378] -> w371
          tunnel: w367 -> [w380]
          tunnel: w366 -> [w379]
          frame #0 {
            n206 = call "Sync scrollbars.vi"("Min cursor moved"=w374, "Scrollbar value"=w375) -> ()  [unwired: 9 in, 1 out]
          }
          frame #1 {
            n207 = call "Event case-Scrollbar value change.vi"("Tick count in"=w380, "Queue in"=w379) -> ("Tick count"=w378:u32)  [unwired: 8 in, 1 out]
          }
        }
      }
      event "Colour": Value Change {
        n208 = event-data() -> ()  [unwired: 1 in, 1 out]
        n209 = call "Prepare image colour.vi"("Left Image Palette"="Colour") -> ("Color Palette"=w382:cluster{"Red":u8, "Green":u8, "Blue":u8}[], "Palette Type"=w383:u32)  [unwired: 8 in, 1 out]
        n210 = property on="Image" class="ImageControl"("Palette Type"=w383, "User Palette"=w382) -> ()  [unwired: 2 in, 2 out]
      }
      event "Experiment path": Value Change {
        n211 = event-data() -> ()  [unwired: 1 in, 1 out]
        n212 = Enqueue Element At Opposite End(queue=w389, element=Speed_Viewer_States_enum."Initialise") -> ()  [unwired: 2 in, 3 out]
        n213 = local write "Stop"(TRUE ("Stop")) -> ()
      }
      event "Speed chart history (sec)": Value Change {
        n214 = event-data() -> ()  [unwired: 1 in, 1 out]
        n215 = call "Volume img-Init speed chart history.vi"() -> ()  [unwired: 11 in, 1 out]
      }
      event "Cams.Vid 1", "Cams.Vid 2", "Cams.Vid 3", "Cams.Vid 4": Mouse Down {
        # "http://zone.ni.com/reference/en-XX/help/371361K-01/lvhowto/drag_and_drop_programmatic_prepare/"
        # "Detects and registers when the mouse is clicked \nwithin the boundaries of a CamVid display. This allows to generate a \"Drag leave\" event for those displays (in a separate event case / Mouse leave case).\nThis is necessary because the Drag-Leave event does not work for this type of control."
        n216 = event-data() -> ("Button"=w394:u16, "Mods.Double Click"=w396:bool, "CtlRef"=w395:refnum<vi>)  [unwired: 1 in]
        n217 = case shown="True" w396 {
          tunnel: w394 -> [_ w399]
          tunnel: w395 -> [_ w401]
          frame False {
          }
          frame True {
            n218 = property class="ImageControl"(reference=w401) -> ("Label.Text"=w400:string)  [unwired: 1 in, 2 out]
            n219 = call "Open expanded image window.vi"("Button"=w399, "Image name"=w400) -> ()  [unwired: 10 in]
          }
        }
        n220 = case shown="1" w394 {
          tunnel: [_ TRUE] -> w393
          frame 0, Default {
          }
          frame 1 {
          }
        }
      }
      event "Cams.Vid 1", "Cams.Vid 2", "Cams.Vid 3", "Cams.Vid 4": Mouse Leave {
        n221 = event-data() -> ("CtlRef"=w402:refnum<vi>)  [unwired: 1 in]
        n222 = case shown="True" w404 {
          tunnel: w402 -> [_ w408]
          frame False {
          }
          frame True {
            n223 = property class="ImageControl"(reference=w408) -> ("Label.Text"=w406:string)  [unwired: 1 in, 2 out]
            n224 = call "Open expanded image window.vi"("Button"=u16 0, "Image name"=w406) -> ()  [unwired: 10 in]
          }
        }
      }
      event Mouse Up {
        n225 = event-data() -> ()  [unwired: 1 in, 1 out]
      }
      event "Back": Value Change {
        n226 = event-data() -> ()  [unwired: 1 in, 1 out]
        n227 = Enqueue Element At Opposite End(queue=w412, element=Speed_Viewer_States_enum."Back to start") -> ()  [unwired: 2 in, 3 out]
        n228 = local write "Stop"(TRUE ("Stop")) -> ()
      }
      event Value Change {
        n229 = event-data() -> ()  [unwired: 1 in, 1 out]
        n230 = call "16-bit display mapping.vi"() -> (2:w417)  [unwired: 10 in, 1 out]
        n231 = property on="Image" class="ImageControl"("16-bit Display Mapping"=w417) -> ()  [unwired: 2 in, 2 out]
      }
      event "Play": Value Change {
        n232 = event-data() -> ()  [unwired: 1 in, 1 out]
        n233 = flat-sequence {
          tunnel: w422 -> [w426]
          tunnel: [w426] -> w421
          tunnel: w421 -> [w427]
          tunnel: [w427] -> w420
          tunnel: w420 -> [w428]
          frame #0 {
            n234 = local write "Stop"(FALSE ("Stop")) -> ()
            n235 = call "Set Play-Stop buttons.vi"("Function"=Select_Play-Stop_button_to_show."Show Stop button") -> ()  [unwired: 10 in, 1 out]
          }
          frame #1 {
          }
          frame #2 {
            n236 = Enqueue Element(queue=w428, element=Speed_Viewer_States_enum."Playback" ("States")) -> ()  [unwired: 2 in, 3 out]
          }
        }
      }
      event "Stop": Value Change {
        n237 = event-data() -> ()  [unwired: 1 in, 1 out]
      }
      event Panel Close? {
        # "The panel close is always discarded here because it is closed conditionally in the yellow \"Save Windows Bounds\" vi."
        n238 = event-data() -> ()  [unwired: 1 in, 1 out]
        n239 = call "Time series viewer-Event handler-Exit.vi"("Queue in"=w437) -> ("Exit"=w436:bool)  [unwired: 10 in]
        n240 = case shown="True" w436 {
          frame False {
          }
          frame True {
            n241 = local write "Stop"(TRUE ("Stop")) -> ()
            n242 = global write "gl_Time series viewer globals.vi" "Close larger image windows"(TRUE ("Close larger image window")) -> ()
          }
        }
        n243 = property class="VI"(reference=w433) -> ("FP.State"=w434:T20)  [unwired: 1 in, 2 out]
        n244 = event-data("Discard?"=TRUE) -> ()  [unwired: 1 in, 1 out]
      }
    }
  }
  n245 = disable-structure shown="Disabled" {
    frame Disabled {
      # "AVI1 VIs"
      n246 = call "IMAQ AVI Create"() -> ()  [unwired: 10 in, 2 out]
      n247 = call "IMAQ AVI Open"() -> ()  [unwired: 10 in, 2 out]
      n248 = call "IMAQ AVI Read Frame"() -> ()  [unwired: 8 in, 4 out]
      n249 = call "IMAQ AVI Write Frame"() -> ()  [unwired: 10 in, 2 out]
      n250 = call "IMAQ AVI Get Info"() -> ()  [unwired: 7 in, 5 out]
      n251 = call "IMAQ AVI Close"() -> ()  [unwired: 11 in, 1 out]
    }
    frame Enabled {
    }
  }
  n252 = call "Save_Windows_Bounds.vi"("FP.State"=w4, "Window Name (i.e. Key)"=w9, "Front Panel Window:Open"=TRUE, "Window VI's Ref"=w6) -> ()  [unwired: 7 in, 1 out]
  n253 = call "AVI-Viewer cleanup.vi"("error in (no error)"=w27, "RGB image ref"=w18, "I16 image ref"=w32) -> ()  [unwired: 8 in, 1 out]
